vi "PixmapWrite.vi"(0 "Pixmap.bin path":path, 2 "Depth":i32, 3 "Width":i16, 4 "Height":i16, 5 "Pixels colors (CLUT)":u8[](array[numeric]), 7 "PNGFile error":errorcluster) -> (13 "Pixmap.bin error":errorcluster)   [LabVIEW 2023]
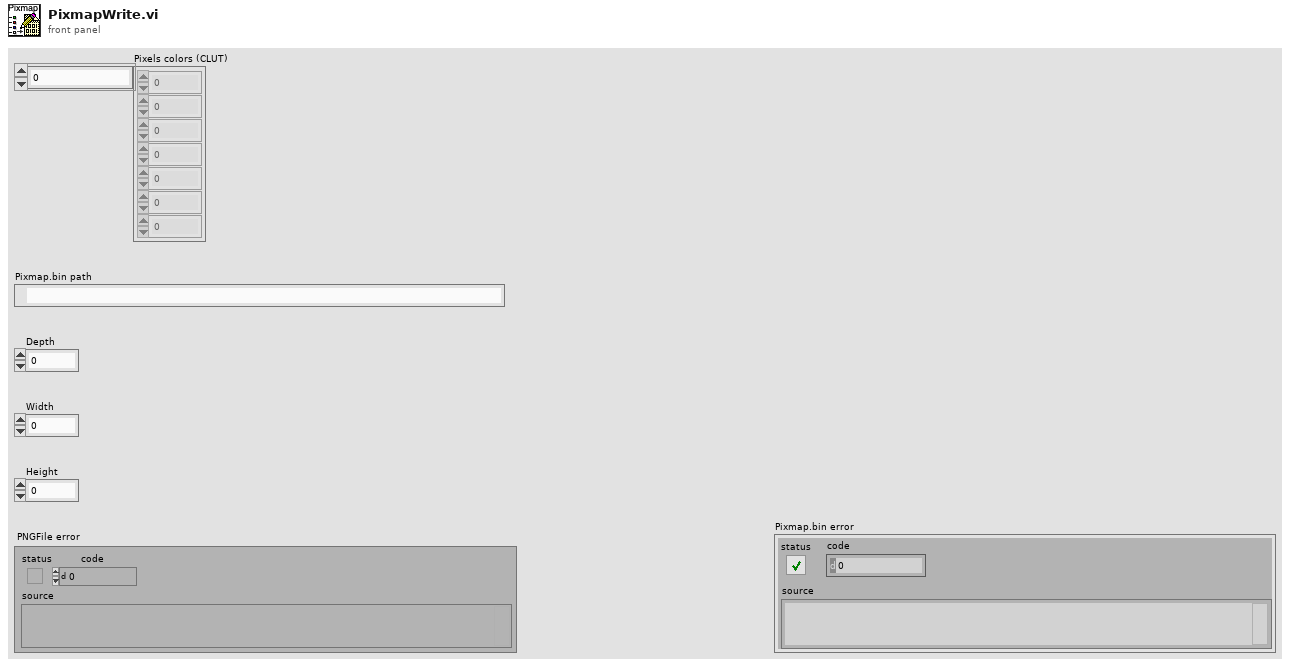
[diagram p1: front panel]
types:
  T1 = enum16{"big-endian, network order", "native, host order", "little-endian"}
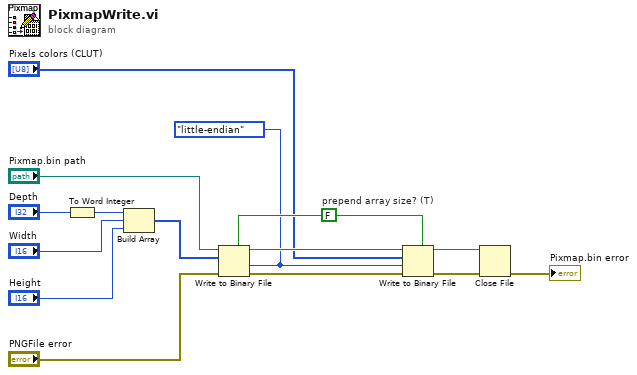
[diagram p0: block diagram]
diagram:
  w8 = T1."little-endian" ("byte order (0:big-endian, network order)")
  w9 = FALSE  # prepend array size? (T)
  n1 = To Word Integer(number="Depth") -> (16bit integer=w12:i16)
  n2 = Build Array(w12, "Width", "Height") -> (w10:i16[])
  n3 = Write to Binary File(file (use dialog)="Pixmap.bin path", data=w10, error in="PNGFile error", 5:w9, 9:w8) -> (refnum out=w13:refnum<file>, error out=w6:errorcluster)  [unwired: 1 in, 1 out]
  n4 = Write to Binary File(file (use dialog)=w13, data="Pixels colors (CLUT)", error in=w6, 5:w9, 9:w8) -> (refnum out=w15:refnum<file>, error out=w14:errorcluster)  [unwired: 1 in, 1 out]
  n5 = Close File(refnum=w15, error in=w14) -> (error out=→"Pixmap.bin error":errorcluster)  [unwired: 1 out]
